vi "SeCrTS-Obtain notifier display.vi"(8 "error in (no error)":errorcluster) -> (0 "error out":errorcluster, 3 "NOT DIS Out":T1)   [LabVIEW 2022 SP3]
uses:
  Control/SeCrTS-Notifier Ref.ctl
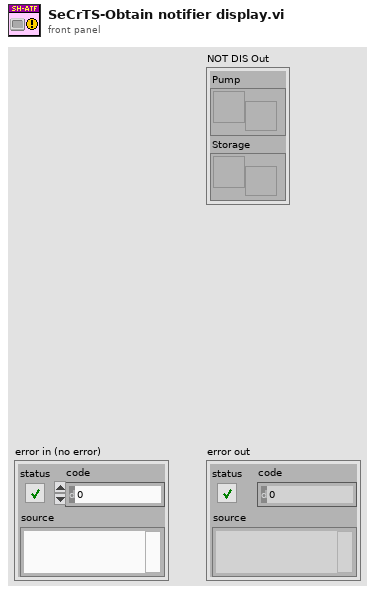
[diagram p1: front panel]
types:
  T1 = typedef "SeCrTS-Notifier Ref.ctl" = cluster{"Pump":refnum<notifier>, "Storage":refnum<notifier>}
  T2 = cluster{"AI_V_Data":waveform(dbl)[][], "DO_Data":waveform(dbl)[][], "DI_Data":digitalwaveform[][]}
  T3 = cluster{"AI_V_Data":waveform(dbl)[][], "AI_C_Data":waveform(dbl)[][], "AO_Data":waveform(dbl)[][], "DO_Data":waveform(dbl)[][], "DI_Data":digitalwaveform[][], "ACC_Data":waveform(dbl)[][], "TC Data":waveform(dbl)[][], "Drive_A_C":waveform(dbl)[][], "Drive_A_D":waveform(dbl)[][], "AI_V Rms":waveform(dbl)[][]}
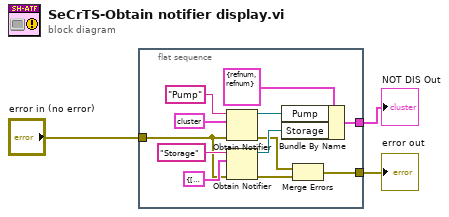
[diagram p0: block diagram]
diagram:
  n1 = flat-sequence {
    tunnel: "error in (no error)" -> [w7]
    tunnel: [w4] -> w2
    tunnel: [w11] -> w1
    frame #0 {
      n2 = Obtain Notifier(name (unnamed)="Pump", notification data type=T3 data[101840B] ("data out 2"), error in (no error)=w7) -> (notifier out=w12:refnum<notifier>, error out=w6:errorcluster)  [unwired: 1 in, 1 out]
      n3 = Obtain Notifier(name (unnamed)="Storage", notification data type=T2 {"AI_V_Data"=[], "DO_Data"=[], "DI_Data"=[]} ("value"), error in (no error)=w7) -> (notifier out=w8:refnum<notifier>, error out=w5:errorcluster)  [unwired: 1 in, 1 out]
      n4 = Bundle By Name(cluster=T1 {"Pump"=refnum, "Storage"=refnum} ("NOT DIS Out"), "Pump"=w12, "Storage"=w8) -> (w11:T1)
      n5 = Merge Errors(w6, w5) -> (w4:errorcluster)
    }
  }
  "error out" <- w2
  "NOT DIS Out" <- w1
